vi "测量流程.vi"(11 "控制命令":T1(ring)) -> ()   [LabVIEW 2016, in "斯坦道总氮V2.lvlib"]
panel:
  out "x-y":dbl
  out "当前时间":timestamp
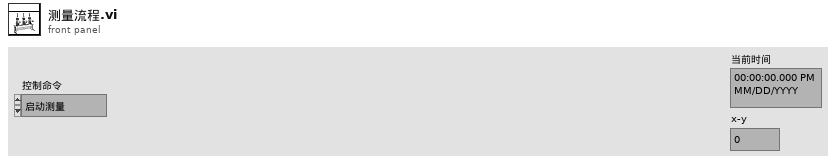
[diagram p1: front panel]
types:
  T1 = enum16{"启动测量", "标样核查", "零点核查", "跨度核查", "空白测试", "平行样测试", "加标回收", "空白校准", "标样校准", "初始化（清洗）", "停止测试", "仪器重启", "校时", "模式设置", "测量间隔设置"}
  T2 = cluster{"站号":u16, "量程切换":enum32{"H", "L", "AUTO"}, "控制命令":enum16{"启动测量", "标样核查", "零点核查", "跨度核查", "空白测试", "平行样测试", "加标回收", "空白校准", "标样校准", "初始化（清洗）", "停止测试", "仪器重启", "校时", "模式设置", "测量间隔设置"}, "模式设置":enum16{"待机", "连续模式", "周期模式", "定点模式", "受控模式", "手动模式"}, "测量间隔":u16}
  T3 = cluster{"时间标识":timestamp, "设备":string, "日志信息":string, "流程参数":string}
  T4 = enum16{"空闲", "水样测试", "标样核查", "零点核查", "跨度核查", "空白测试", "平行样测试", "加标回收", "空白校准", "标样校准", "初始化（清洗）"}
  T5 = cluster{"系统时间":timestamp, "工作状态":u16, "测量模式":enum16{"待机", "连续模式", "周期模式", "定点模式", "受控模式", "手动模式"}, "告警代码":u16, "故障代码":u16, "日志代码":u16, "软件版本":u16, "F0":sgl, "F1":sgl, "F2":sgl, "F3":sgl, "T":sgl, "H":sgl, "id":u16, "flowid":u16, "量程":u16, "总磷控温温度1":sgl, "营养盐控温温度2":sgl, "ADC":sgl}
  T6 = cluster{"水样测试量程模式":enum16{"H", "L", "AUTO"}, "空白核查量程模式":enum16{"H", "L", "AUTO"}, "跨度核查量程模式":enum16{"H", "L", "AUTO"}, "加标回收量程模式":enum16{"H", "L", "AUTO"}, "标样核查量程模式":enum16{"H", "L", "AUTO"}}
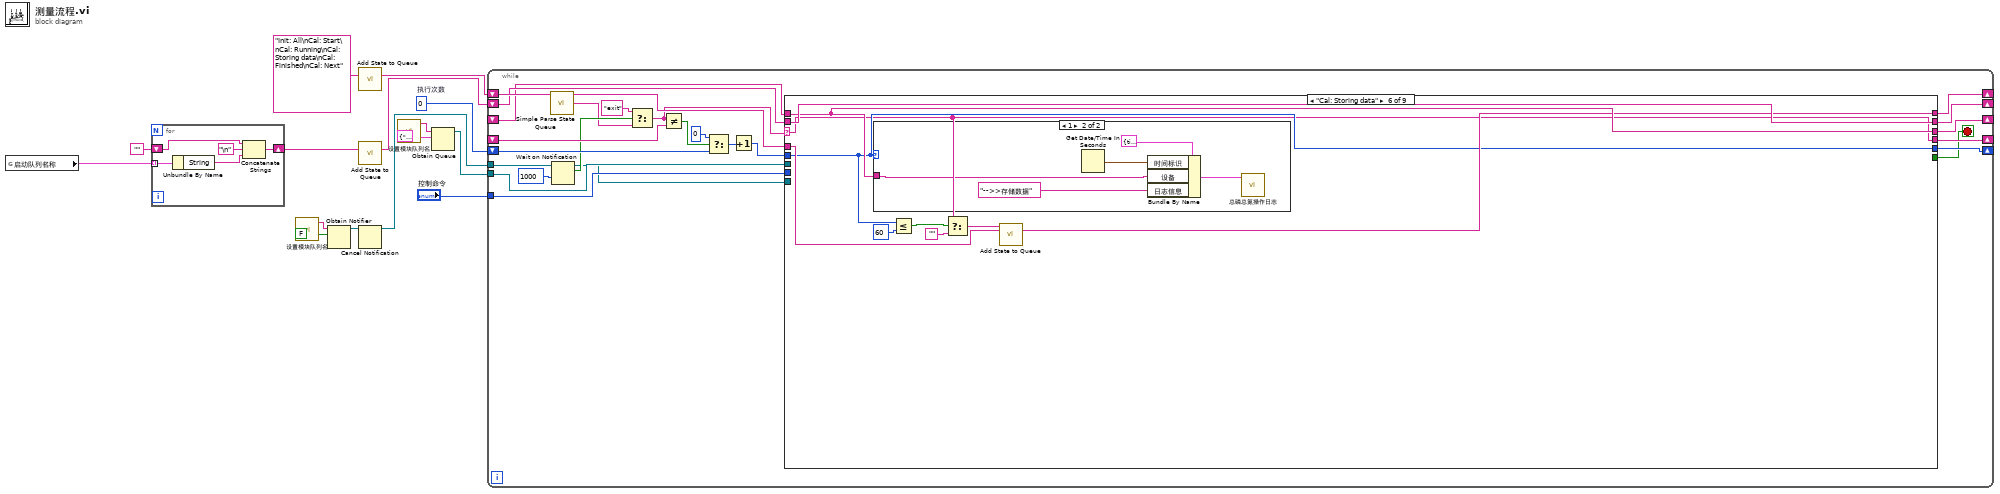
[diagram p0: block diagram]
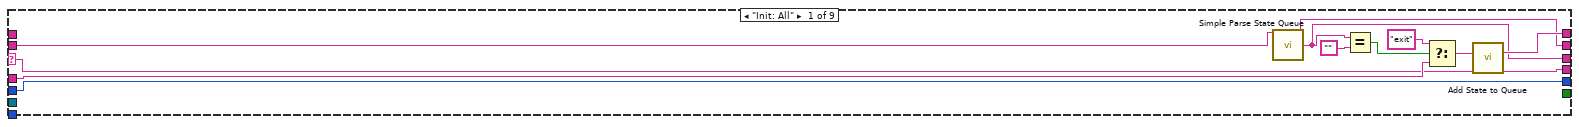
[diagram p2: hidden frame]
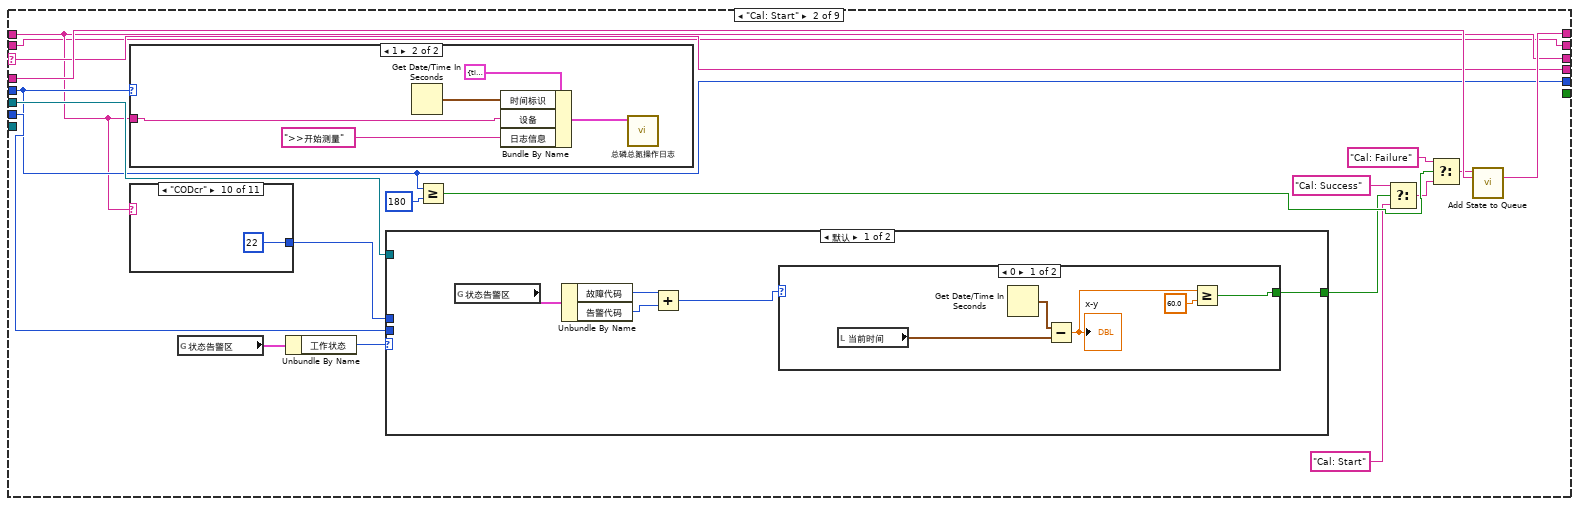
[diagram p3: hidden frame]
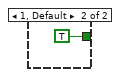
[diagram p4: hidden frame]
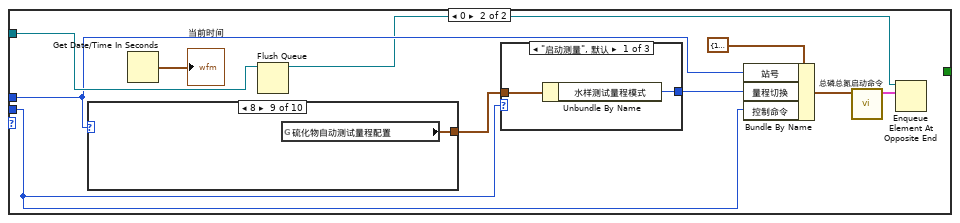
[diagram p5: hidden frame]
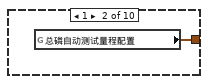
[diagram p7: hidden frame]
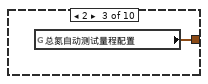
[diagram p8: hidden frame]
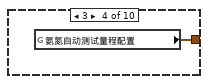
[diagram p9: hidden frame]
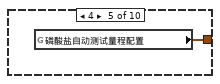
[diagram p10: hidden frame]
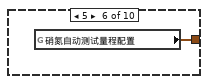
[diagram p11: hidden frame]
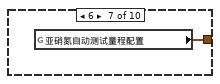
[diagram p12: hidden frame]
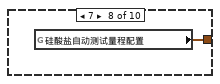
[diagram p13: hidden frame]
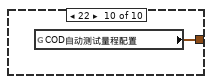
[diagram p14: hidden frame]
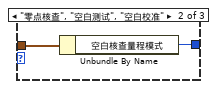
[diagram p15: hidden frame]
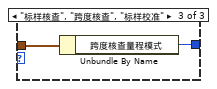
[diagram p16: hidden frame]
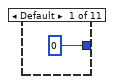
[diagram p17: hidden frame]
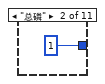
[diagram p18: hidden frame]
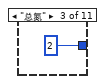
[diagram p19: hidden frame]
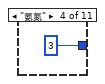
[diagram p20: hidden frame]
diagram:
  w9 = 0  # 执行次数
  n1 = global read "总磷总氮断电保存全局变量.vi" "启动队列名称"() -> (w1:cluster{"String":string, "Value":u16}[])
  n2 = for {
    shift-right: [w19] -> w2
    shift-left: "" -> [w20]
    tunnel: w1 -> [w18] mode=indexing
    n3 = Unbundle By Name(w18) -> ("String"=w17:string)
    n4 = Concatenate Strings(w20, "\n", w17) -> (w19:string)
  }
  n5 = call "设置模块队列名.vi"() -> ("Msg"=w6:string)  [unwired: 5 in]
  n6 = Obtain Notifier(name (unnamed)=w6, notification data type=FALSE) -> (notifier out=w14:refnum<notifier>)  [unwired: 2 in, 2 out]
  n7 = call "Add State to Queue.vi"("State(s) In (\"\")"="Init: All\nCal: Start\nCal: Running\nCal: Storing data\nCal: Finished\nCal: Next" ("State(s) In (\"\")")) -> ("States Out"=w12:string)  [unwired: 14 in]
  n8 = call "Add State to Queue.vi"("State(s) In (\"\")"=w2) -> ("States Out"=w7:string)  [unwired: 14 in]
  n9 = Cancel Notification(0:w14) -> (8:w4:refnum<notifier>)  [unwired: 1 in, 2 out]
  n10 = call "设置模块队列名.vi"() -> ("Msg"=w5:string)  [unwired: 5 in]
  n11 = Obtain Queue(name (unnamed)=w5, element data type=cluster{"命令":string, "data":variant} {"命令"="", "data"=variant}) -> (queue out=w10:refnum<queue>)  [unwired: 3 in, 2 out]
  n12 = while {
    tunnel: w10 -> [w43]
    shift-right: [w42] -> _
    shift-left: w12 -> [w45]
    shift-right: [w35] -> _
    shift-left: w9 -> [w38]
    shift-right: [w41] -> _
    shift-left: _ -> [w40]
    tunnel: "控制命令" -> [w33]
    shift-right: [w29] -> _
    shift-left: w7 -> [w31]
    shift-right: [w30] -> _
    shift-left: _ -> [w28]
    tunnel: w4 -> [w26]
    stop <- w32 stop-if-true
    n13 = call "Simple Parse State Queue.vi"("State Queue"=w45) -> ("Remain States"=w44:string, "Next State"=w23:string)  [unwired: 13 in]
    n14 = Wait on Notification(notifier=w26, timeout in ms (-1)=1000 ("超时毫秒(-1)")) -> (notifier out=w21:refnum<notifier>, notification=w25:bool)  [unwired: 2 in, 2 out]
    n15 = Select(t="exit", s=w25, f=w23) -> (s? t:f=w22:string)
    n16 = Not Equal?(x=w22, y=w40) -> (x != y?=w39:bool)
    n17 = Select(t=0, s=w39, f=w38) -> (s? t:f=w36:i32)
    n18 = Increment(x=w36) -> (x+1=w34:i32)
    n19 = case shown="\"Cal: Storing data\"" w22 {
      selector: w22 -> [w52 w73 w131 w146 w152 w166 w182 w193 w200]
      tunnel: w44 -> [w54 w75 w133 _ w163 w171 w184 _ w201]
      tunnel: w43 -> [_ w71 _ _ _ _ _ _ w196]
      tunnel: [w56 w74 w132 w147 w162 w170 w183 "Init: All\nCal: Start\nCal: Running\nCal: Storing data\nCal: Finished\nCal: Next" ("State(s) In (\"\")") w201] -> w42
      tunnel: [w52 w73 w131 w146 w152 w166 w182 w193 w200] -> w41
      tunnel: [w51 w68 w130 w145 w155 w169 w180 w192 w199] -> w35
      tunnel: w34 -> [w51 w68 w130 w145 w155 w169 w180 w192 w199]
      tunnel: w33 -> [_ w70 _ _ _ _ _ _ _]
      tunnel: [_ _ _ _ _ _ _ _ TRUE] -> w32
      tunnel: w31 -> [w50 w57 w129 w139 w149 w173 w181 w191 w198]
      tunnel: [w48 w58 w128 w138 w148 w172 w179 w190 w197] -> w30
      tunnel: [w49 w57 w129 w139 w149 w173 w181 w191 w198] -> w29
      tunnel: w28 -> [_ w58 w128 w138 w148 w172 w179 w190 w197]
      tunnel: w21 -> [_ _ _ _ _ _ _ _ w195]
      frame "Init: All" {
        n20 = call "Simple Parse State Queue.vi"("State Queue"=w50) -> ("Remain States"=w49:string, "Next State"=w48:string)  [unwired: 13 in]
        n21 = Equal?(x=w48, y="") -> (x = y?=w46:bool)
        n22 = Select(t="exit", s=w46, f=w54) -> (s? t:f=w53:string)
        n23 = call "Add State to Queue.vi"("State(s) In (\"\")"=w53) -> ("States Out"=w56:string)  [unwired: 14 in]
      }
      frame "Cal: Start" {
        n24 = case shown="1" w68 {
          tunnel: w58 -> [_ w123]
          frame 0, Default {
          }
          frame 1 {
            n25 = Get Date/Time In Seconds() -> (seconds since 1Jan1904=w127:timestamp)
            n26 = Bundle By Name(cluster=T3 {"时间标识"=timestamp(0 s since 1904-01-01), "设备"="", "日志信息"="", "流程参数"=""} ("data in"), "时间标识"=w127, "设备"=w123, "日志信息"=">>开始测量") -> (w126:T3)
            n27 = call "总磷总氮操作日志.vi"("data in"=w126) -> ()  [unwired: 10 in, 1 out]
          }
        }
        n28 = case shown="\"CODcr\"" w58 {
          tunnel: [0 1 2 3 4 5 6 7 8 22 22] -> w69
          frame Default {
          }
          frame "总磷" {
          }
          frame "总氮" {
          }
          frame "氨氮" {
          }
          frame "磷酸盐" {
          }
          frame "硝氮" {
          }
          frame "亚硝氮" {
          }
          frame "硅酸盐" {
          }
          frame "硫化物" {
          }
          frame "CODcr" {
          }
          frame "COD" {
          }
        }
        n29 = global read "VAR总磷总氮全局变量.vi" "状态告警区"() -> (w72:T5)
        n30 = Unbundle By Name(w72) -> ("工作状态"=w59:u16)
        n31 = case shown="默认" w59 {
          tunnel: w70 -> [_ w92]
          tunnel: w71 -> [_ w95]
          tunnel: [w80 _] -> w63
          tunnel: w69 -> [_ w90]
          frame Default {
            n32 = global read "VAR总磷总氮全局变量.vi" "状态告警区"() -> (w79:T5)
            n33 = Unbundle By Name(w79) -> ("故障代码"=w77:u16, "告警代码"=w78:u16)
            n34 = Add(x=w77, y=w78) -> (x+y=w76:u16)
            n35 = case shown="0" w76 {
              tunnel: [w81 TRUE] -> w80
              frame 0 {
                n36 = local read "当前时间"() -> (w85:timestamp)
                n37 = Get Date/Time In Seconds() -> (seconds since 1Jan1904=w84:timestamp)
                n38 = Subtract(x=w84, y=w85) -> (x-y=w83:dbl)
                "x-y" <- w83
                n39 = Greater Or Equal?(x=w83, y=60.0) -> (x >= y?=w81:bool)
              }
              frame 1, Default {
              }
            }
          }
          frame 0 {
            n40 = case shown="8" w90 {
              tunnel: [_ w97 w98 w99 w100 w101 w102 w103 w104 w105] -> w91
              frame 0, Default {
              }
              frame 1 {
                n41 = global read "总磷总氮断电保存全局变量.vi" "总磷自动测试量程配置"() -> (w97:T6)
              }
              frame 2 {
                n42 = global read "总磷总氮断电保存全局变量.vi" "总氮自动测试量程配置"() -> (w98:T6)
              }
              frame 3 {
                n43 = global read "总磷总氮断电保存全局变量.vi" "氨氮自动测试量程配置"() -> (w99:T6)
              }
              frame 4 {
                n44 = global read "总磷总氮断电保存全局变量.vi" "磷酸盐自动测试量程配置"() -> (w100:T6)
              }
              frame 5 {
                n45 = global read "总磷总氮断电保存全局变量.vi" "硝氮自动测试量程配置"() -> (w101:T6)
              }
              frame 6 {
                n46 = global read "总磷总氮断电保存全局变量.vi" "亚硝氮自动测试量程配置"() -> (w102:T6)
              }
              frame 7 {
                n47 = global read "总磷总氮断电保存全局变量.vi" "硅酸盐自动测试量程配置"() -> (w103:T6)
              }
              frame 8 {
                n48 = global read "总磷总氮断电保存全局变量.vi" "硫化物自动测试量程配置"() -> (w104:T6)
              }
              frame 22 {
                n49 = global read "总磷总氮断电保存全局变量.vi" "COD自动测试量程配置"() -> (w105:T6)
              }
            }
            n50 = Get Date/Time In Seconds() -> (seconds since 1Jan1904=→"当前时间":timestamp)
            n51 = Flush Queue(queue=w95) -> (queue out=w88:refnum<queue>)  [unwired: 1 in, 2 out]
            n52 = case shown="\"启动测量\", 默认" w92 {
              tunnel: w91 -> [w107 w109 w111]
              tunnel: [w106 w108 w110] -> w96
              frame "启动测量", Default {
                n53 = Unbundle By Name(w107) -> ("水样测试量程模式"=w106:enum16{"H", "L", "AUTO"})
              }
              frame "零点核查", "空白测试", "空白校准" {
                n54 = Unbundle By Name(w109) -> ("空白核查量程模式"=w108:enum16{"H", "L", "AUTO"})
              }
              frame "标样核查", "跨度核查", "标样校准" {
                n55 = Unbundle By Name(w111) -> ("跨度核查量程模式"=w110:enum16{"H", "L", "AUTO"})
              }
            }
            n56 = Bundle By Name(cluster=T2 {"站号"=1, "量程切换"=enum."AUTO", "控制命令"=enum."启动测量", "模式设置"=enum."待机", "测量间隔"=0} ("参数"), "站号"=w90, "量程切换"=w96, "控制命令"=w92) -> (w93:T2)
            n57 = call "总磷总氮启动命令.vi"("参数"=w93) -> ("启动命令"=w89:cluster{"命令":string, "data":variant})  [unwired: 10 in]
            n58 = Enqueue Element At Opposite End(queue=w88, element=w89) -> ()  [unwired: 2 in, 3 out]
          }
        }
        n59 = Greater Or Equal?(x=w68, y=180) -> (x >= y?=w66:bool)
        n60 = Select(t="Cal: Success" ("State(s) In (\"\")"), s=w63, f="Cal: Start" ("State(s) In (\"\")")) -> (s? t:f=w61:string)
        n61 = Select(t="Cal: Failure" ("State(s) In (\"\")"), s=w66, f=w61) -> (s? t:f=w64:string)
        n62 = call "Add State to Queue.vi"("State(s) In Front (\"\")"=w64, "State(s) In (\"\")"=w75) -> ("States Out"=w74:string)  [unwired: 13 in]
      }
      frame "Cal: Success" {
        n63 = Get Date/Time In Seconds() -> (seconds since 1Jan1904=w136:timestamp)
        n64 = Bundle By Name(cluster=T3 {"时间标识"=timestamp(0 s since 1904-01-01), "设备"="", "日志信息"="", "流程参数"=""} ("data in"), "时间标识"=w136, "设备"=w128, "日志信息"="-->>启动成功") -> (w135:T3)
        n65 = call "总磷总氮操作日志.vi"("data in"=w135) -> ()  [unwired: 10 in, 1 out]
        n66 = call "Add State to Queue.vi"("State(s) In (\"\")"=w133) -> ("States Out"=w132:string)  [unwired: 14 in]
      }
      frame "Cal: Failure" {
        n67 = Get Date/Time In Seconds() -> (seconds since 1Jan1904=w143:timestamp)
        n68 = Bundle By Name(cluster=T3 {"时间标识"=timestamp(0 s since 1904-01-01), "设备"="", "日志信息"="", "流程参数"=""} ("data in"), "时间标识"=w143, "设备"=w138, "日志信息"="-->>启动失败") -> (w142:T3)
        n69 = call "总磷总氮操作日志.vi"("data in"=w142) -> ()  [unwired: 10 in, 1 out]
        n70 = call "Add State to Queue.vi"("State(s) In (\"\")"="exit" ("State(s) In (\"\")")) -> ("States Out"=w147:string)  [unwired: 14 in]
      }
      frame "Cal: Running" {
        n71 = global read "VAR总磷总氮全局变量.vi" "状态告警区"() -> (w159:T5)
        n72 = Less Or Equal?(x=w155, y=7200) -> (x <= y?=w153:bool)
        n73 = Unbundle By Name(w159) -> ("工作状态"=w160:u16)
        n74 = Select(t=w152, s=w153, f="exit") -> (s? t:f=w151:string)
        n75 = Equal?(x=w160, y=T4."空闲") -> (x = y?=w158:bool)
        n76 = Select(t="", s=w158, f=w151) -> (s? t:f=w156:string)
        n77 = call "Add State to Queue.vi"("State(s) In Front (\"\")"=w156, "State(s) In (\"\")"=w163) -> ("States Out"=w162:string)  [unwired: 13 in]
      }
      frame "Cal: Storing data" {
        n78 = case shown="1" w169 {
          tunnel: w172 -> [_ w174]
          frame 0, Default {
          }
          frame 1 {
            n79 = Get Date/Time In Seconds() -> (seconds since 1Jan1904=w178:timestamp)
            n80 = Bundle By Name(cluster=T3 {"时间标识"=timestamp(0 s since 1904-01-01), "设备"="", "日志信息"="", "流程参数"=""} ("data in"), "时间标识"=w178, "设备"=w174, "日志信息"="-->>存储数据") -> (w177:T3)
            n81 = call "总磷总氮操作日志.vi"("data in"=w177) -> ()  [unwired: 10 in, 1 out]
          }
        }
        n82 = Less Or Equal?(x=w169, y=60) -> (x <= y?=w167:bool)
        n83 = Select(t=w166, s=w167, f="") -> (s? t:f=w164:string)
        n84 = call "Add State to Queue.vi"("State(s) In Front (\"\")"=w164, "State(s) In (\"\")"=w171) -> ("States Out"=w170:string)  [unwired: 13 in]
      }
      frame "Cal: Finished" {
        n85 = case shown="1" w180 {
          tunnel: w179 -> [_ w185]
          frame 0, Default {
          }
          frame 1 {
            n86 = Get Date/Time In Seconds() -> (seconds since 1Jan1904=w189:timestamp)
            n87 = Bundle By Name(cluster=T3 {"时间标识"=timestamp(0 s since 1904-01-01), "设备"="", "日志信息"="", "流程参数"=""} ("data in"), "时间标识"=w189, "设备"=w185, "日志信息"="测量结束>>") -> (w188:T3)
            n88 = call "总磷总氮操作日志.vi"("data in"=w188) -> ()  [unwired: 10 in, 1 out]
          }
        }
        n89 = call "Add State to Queue.vi"("State(s) In (\"\")"=w184) -> ("States Out"=w183:string)  [unwired: 14 in]
      }
      frame "Cal: Next" {
      }
      frame "exit", Default {
        n90 = Release Queue(queue=w196) -> ()  [unwired: 2 in, 3 out]
        n91 = Release Notifier(notifier=w195) -> ()  [unwired: 2 in, 3 out]
      }
    }
  }
